vi "Parse Formula Variables.vi"(11 "Formula":string) -> (3 "Variables":string[](array[string]))   [LabVIEW 2019, in "Simple SysDef API.lvlib"]
uses:
  <userlib>/SimpleSysDef/Simple SysDef API.lvlib
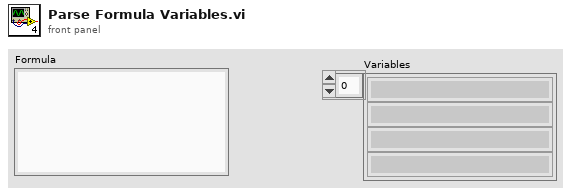
[diagram p1: front panel]
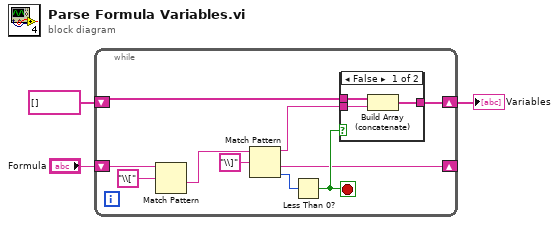
[diagram p0: block diagram]
diagram:
  n1 = while {
    shift-right: [w12] -> w1
    shift-left: string[] [] -> [w13]
    shift-right: [w5] -> _
    shift-left: "Formula" -> [w9]
    stop <- w11 stop-if-true
    n2 = Match Pattern(string=w9, regular expression="\\[") -> (after substring=w7:string)  [unwired: 1 in, 3 out]
    n3 = Match Pattern(string=w7, regular expression="\\]") -> (before substring=w6:string, after substring=w5:string, offset past match=w4:i32)  [unwired: 1 in, 1 out]
    n4 = Less Than 0?(x=w4) -> (x < 0?=w11:bool)
    n5 = case shown="False" w11 {
      tunnel: w13 -> [w16 w17]
      tunnel: [w15 w17] -> w12
      tunnel: w6 -> [w14 _]
      frame False {
        n6 = Build Array (concatenate)(w16, w14) -> (w15:string[])
      }
      frame True {
      }
    }
  }
  "Variables" <- w1
